vi "Dashboard Main.vi"() -> ()   [LabVIEW 2016]
uses:
  <vilib>/Utility/miscctls.llb/LVRowAndColumnTypeDef.ctl
  <vilib>/event_ctls.llb/eventvkey.ctl
  <vilib>/Rock Robotics/Network Tables/NT Write Boolean.vi
  <vilib>/Rock Robotics/Network Tables/NT Read Numeric Array.vi
  <vilib>/Rock Robotics/WPI/Dashboard/WPI_DashboardLogging Global.vi
panel:
  out "Camera Image":T1(plugin-control)
  in  "Camera Settings Right":T2={"Frame Rate"=30, "Compression"=30, "Size"=1, "DB Camera Config"=FALSE} {"Frame Rate" scale=1.0..30.0; "Compression" scale=100.0..-1.0; "Size" items=["640x480", "320x240", "160x120"]}
  in  "Camera Name Right":string(combo)="No Camera Selection"
  out "Camera Info":cluster{"Mbps LED":bool, "Mbps":dbl, "fps":dbl} {"fps" format="%#.1g"; "Mbps" format="%#.1g"}
  in  "Camera Settings":T2={"Frame Rate"=30, "Compression"=30, "Size"=1, "DB Camera Config"=FALSE} {"Frame Rate" scale=1.0..30.0; "Compression" scale=100.0..-1.0; "Size" items=["640x480", "320x240", "160x120"]}
  in  "TCP":refnum<k5>
  in  "Rec Mode":enum32{"Stop", "Record", "Playback"}(radio)
  out "Robot IP":string
  out "Image Message":string="Timeout in Camera Communications"
  in  "Dashboard Tab":T3(tab)
  in  "Select Auto":string(combo)="Select Autonomous ..."
  out "NT Connection":bool
  out "MotorChart R":cluster{"Numeric":dbl, "Numeric":dbl}(graph)
  out "MotorChart L":cluster{"Numeric":dbl, "Numeric":dbl}(graph)
  out "MotorSliders R":cluster{"MotorSlide1":dbl, "MotorSlide2":dbl} {"MotorSlide2" scale=-1.0..1.0 scale format="%#_2e"; "MotorSlide1" scale=-1.0..1.0 scale format="%#_2e"}
  out "MotorSliders L":cluster{"MotorSlide1":dbl, "MotorSlide2":dbl} {"MotorSlide2" scale=-1.0..1.0 scale format="%#_2e"; "MotorSlide1" scale=-1.0..1.0 scale format="%#_2e"}
  out "Gyro":dbl(knob) scale=0.0..360.0
  out "JS1 Z":dbl(slide) scale=-1.0..1.0 scale format="%#_2e"
  out "JS1 Graph":cluster{"X":dbl, "Y":dbl}[](graph)
  out "JS1 Buttons":T4
  out "JS2 Z":dbl(slide) scale=-1.0..1.0 scale format="%#_2e"
  out "JS2 Graph":cluster{"X":dbl, "Y":dbl}[](graph)
  out "JS2 Buttons":T4
  out "Mode":T5(ring)=enum."Auto Disabled"
  out "Camera Image Right":T1(plugin-control)
  in  "DB/String 9":string
  in  "DB/String 8":string
  in  "DB/String 7":string
  in  "DB/String 6":string
  in  "DB/String 5":string
  in  "DB/String 4":string
  in  "DB/String 3":string
  in  "DB/String 2":string
  in  "DB/String 1":string
  in  "DB/String 0":string
  in  "DB/Slider 0":dbl(slide) scale=0.0..5.0
  in  "DB/Slider 1":dbl(slide) scale=0.0..5.0
  in  "DB/Slider 2":dbl(slide) scale=0.0..5.0
  in  "DB/Slider 3":dbl(slide) scale=0.0..5.0
  out "DB/LED 3":bool
  out "DB/LED 2":bool
  out "DB/LED 1":bool
  out "DB/LED 0":bool
  in  "DB/Button 3":bool
  in  "DB/Button 2":bool
  in  "DB/Button 1":bool
  in  "DB/Button 0":bool caption="New Name"
  out "2D Picture":picture
  out "String 3 MAGIC":string
  out "Berg Mode":string
  in  "Auton Enabled":bool=TRUE
  out "String 2":string
  out "Steam Power":dbl(knob)=88.16248842081647 scale=0.0..100.0
  in  "Station Loc":T6(radio)
  out "Gyro":dbl(knob) scale=0.0..360.0
  out "Game Time":u8(slide) scale=0.1..100.0
  in  "UpdateCam":bool
  in  "Exposure":dbl(slide) scale=0.0..100.0
  in  "White Bal":dbl(slide) scale=0.0..100.0
  in  "Color Components":T7={"Hue"={110.0, 142.0}, "Sat"={212.5, 255.0}, "Val"={24.285714285714285, 112.32142857142857}, "Boolean"=FALSE} {"Val" scale=0.0..255.0; "Sat" scale=0.0..255.0; "Hue" scale=0.0..255.0 scale format="%#_3g"}
  in  "Camera Mode":u16(ring) items=["Raw", "Interpreted", "Particle", "Paired", "Final"]
  in  "Color Components 2":T7={"Hue"={110.0, 142.0}, "Sat"={212.0, 255.0}, "Val"={24.0, 112.0}, "Boolean"=FALSE} {"Val" scale=0.0..255.0; "Sat" scale=0.0..255.0; "Hue" scale=0.0..255.0 scale format="%#_3g"}
  in  "Camera Mode 2":u16(ring) items=["Raw", "Interpreted", "Particle", "Paired", "Final"]
  in  "Test Slider":dbl(slide) scale=0.0..100.0 scale format="%#_3g"
  in  "On/Off":bool caption="Solenoid"
  in  "Test Name":u16(ring) items=["Select the test to run..."]
  in  "Test Tree":string(tree)
  in  "Motor":cluster{"Value":dbl, "Enable":bool} {"Value" scale=-1.0..1.0 scale format="%#_3g"}
  out "Progress":T8 {"Test Progress" scale=0.0..100.0}
  in  "Rev/Fwd":cluster{"Forward":bool, "Reverse":bool}
  in  "Test Ring":u16(ring) items=["Monochrome", "Color"]
  out "Cmd Status":string
  in  "Execute Command":bool
  in  "Command Params":string[][](table)
  in  "Command Selection":i32(listbox)
  in  "CheckList":i32(listbox)
  out "Tree":string(tree)
  out "Background":bool
  in  "Camera Name":string(combo)="No Camera Selection"
  # "HW"
  # "HW"
  # "Joysticks"
  # "Drive Motors"
  # "Front"
  # "Right"
  # "Left"
  # "Back"
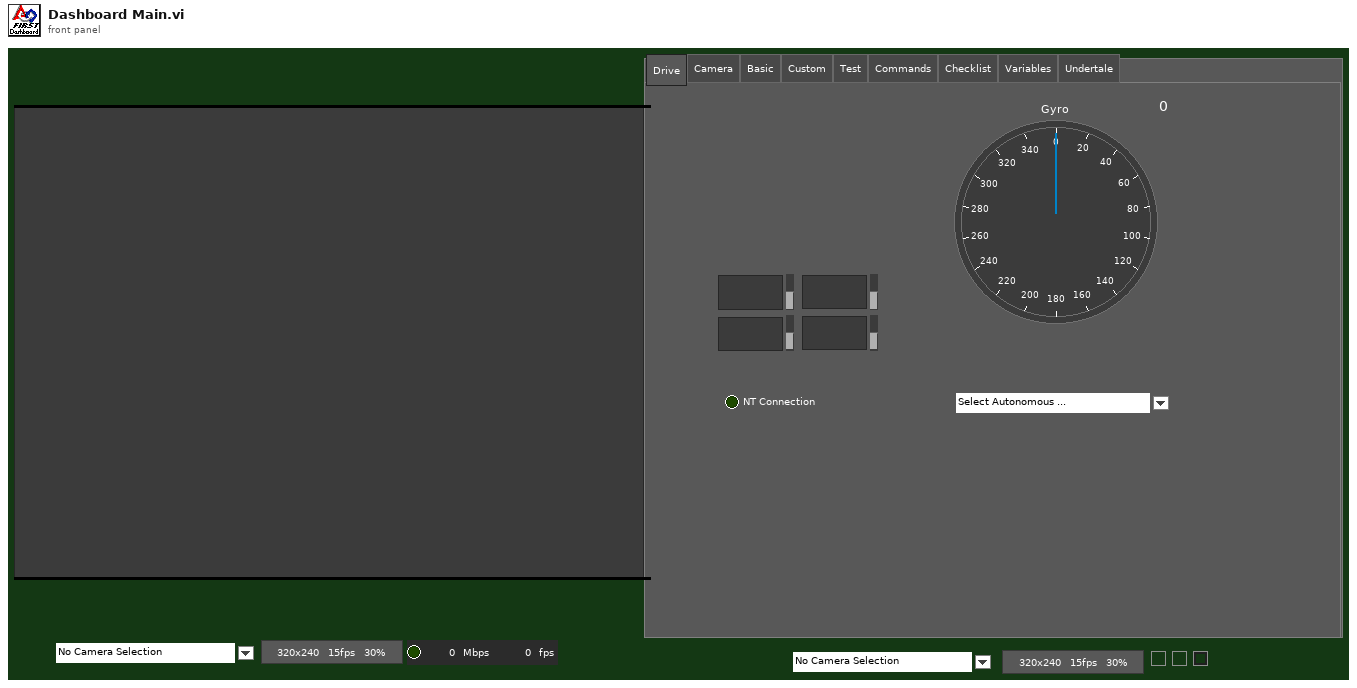
[diagram p1: front panel]
types:
  T1 = typedef "IMAQ Image.ctl" = refnum<image>
  T2 = cluster{"Frame Rate":i32, "Compression":i32, "Size":u16, "DB Camera Config":bool}
  T3 = enum32{"Drive", "Camera", "Basic", "Custom", "Test", "Commands", "Checklist", "Variables", "Undertale"}
  T4 = cluster{bool, bool, bool, bool, bool, bool, bool, bool, bool, bool, bool, bool}
  T5 = enum8{"Tele-Op Disabled", "Tele-Op Enabled", "Auto Disabled", "Auto Enabled", "Test Disabled", "Test Enabled", "Disconnected", "No Code", "E-Stop"}
  T6 = enum32{"Radio Selection 1", "Radio Selection 2", "Radio Selection 3"}
  T7 = cluster{"Hue":cluster{dbl, dbl}, "Sat":cluster{dbl, dbl}, "Val":cluster{dbl, dbl}, "Boolean":bool}
  T8 = cluster{"Test Progress":u8, "Test Progress Text":string}
  T9 = typedef "Image Type" = u32
  T10 = cluster{"IDs":cluster{"RPC field ID":u16, "Unique ID":u16}, "String":string}
  T11 = enum32{"Drive", "Basic", "Custom", "Test", "Checklist", "Variables"}
  T12 = cluster{"Error Strings":string, "Disable Counts":cluster{u16, u16}, "Rail Faults":cluster{u16, u16, u16}, "Robot IP":string, "DB Mode":u8, "Event Info":cluster{"Name":string, "Type":u8, "Number":u16, "Replay":u8}}
  T13 = cluster{"Storage":cluster{"Disk Free":u64, "RAM Block":u32, "RAM free":u32}, "CPU Utilization":cluster{"CPU % ISR":sgl, "CPU % Time Crit":sgl, "CPU % Timed Str":sgl, "CPU % High":sgl, "CPU % Above":sgl, "CPU % Normal":sgl, "CPU % Low":sgl}, "CAN":cluster{"% Bus Utilization":sgl, "Bus Off Cnt":u32, "TX_FIFO Full Cnt":u32, "Receive Error Cnt":u8, "Transmit Error Cnt":u8}, "HID":cluster{"HID Outputs":u32, "Rumble Low":u16, "Rumble High":u16}[]}
  T14 = cluster{"Status bits":cluster{"Test Mode":bool, "Autonomous":bool, "Enabled":bool, "Code Start":bool, "Brownout":bool, "Reserved 2":bool, "Reserved 3":bool, "E-Stop":bool}, "Code Trace":cluster{"Disabled":bool, "TeleOp":bool, "Auto":bool, "Test":bool}, "Controller Type":enum16{"unknown", "cRIO", "roboRio"}, "Code?":enum16{"unknown", "noCode", "code"}, "Battery V":dbl}
  T15 = cluster{"Control Bits":cluster{"TestMode":bool, "Autonomous":bool, "Enabled":bool, "FMS Present":bool, bool, bool, bool, "E-Stop":bool}, "Team Station ":u8, "Countdown":sgl, "Joystick Values":cluster{"Axes":dbl[], "Buttons":bool[], "POVs":i16[]}[]}
  T16 = cluster{"Axes":dbl[], "Buttons":bool[], "POVs":i16[]}[]
  T17 = cluster{"Axes":dbl[], "Buttons":bool[], "POVs":i16[]}
  T18 = cluster{"Buttons[0]":bool, "Buttons[1]":bool, "Buttons[2]":bool, "Buttons[3]":bool, "Buttons[4]":bool, "Buttons[5]":bool, "Buttons[6]":bool, "Buttons[7]":bool, "Buttons[8]":bool, "Buttons[9]":bool, "Buttons[10]":bool, "Buttons[11]":bool}
  T19 = cluster{"Camera Image":refnum<vi>, "Dashboard Tab":refnum<vi>, "Background":refnum<vi>, "Rec Mode":refnum<vi>, "Test Slider":refnum<vi>, "On/Off ":refnum<vi>, "Test Ring":refnum<vi>, "Rev/Fwd":refnum<vi>, "Test Name":refnum<vi>, "Motor":refnum<vi>, "Progress":refnum<vi>, "CheckList":refnum<vi>, "Tree":refnum<vi>, "Test Tree":refnum<vi>, "Command Params":refnum<vi>, "Command Selection":refnum<vi>, "Execute Command":refnum<vi>, "Cmd Status":refnum<vi>, "Camera Settings":refnum<vi>, "Camera Name":refnum<vi>, "Camera Info":refnum<vi>, "Camera Settings Right":refnum<vi>, "Camera Name Right":refnum<vi>, "Camera Image Right":refnum<vi>}
  T20 = cluster{"Target Combined":cluster{"Particle Report":cluster{"Area":dbl, "Number of Holes":dbl, "Bounding Rect":cluster{"Left":dbl, "Top":dbl, "Right":dbl, "Bottom":dbl}, "Center of Mass":cluster{"X":dbl, "Y":dbl}, "Orientation":dbl, "Dimensions":cluster{"Width":dbl, "Height":dbl}}, "Aspect Ratio Score":dbl, "Vertical Hollowness":dbl, "Horizontal Hollowness":dbl}, "Target A":cluster{"Particle Report":cluster{"Area":dbl, "Number of Holes":dbl, "Bounding Rect":cluster{"Left":dbl, "Top":dbl, "Right":dbl, "Bottom":dbl}, "Center of Mass":cluster{"X":dbl, "Y":dbl}, "Orientation":dbl, "Dimensions":cluster{"Width":dbl, "Height":dbl}}, "Aspect Ratio Score":dbl, "Vertical Hollowness":dbl, "Horizontal Hollowness":dbl}, "Target B":cluster{"Particle Report":cluster{"Area":dbl, "Number of Holes":dbl, "Bounding Rect":cluster{"Left":dbl, "Top":dbl, "Right":dbl, "Bottom":dbl}, "Center of Mass":cluster{"X":dbl, "Y":dbl}, "Orientation":dbl, "Dimensions":cluster{"Width":dbl, "Height":dbl}}, "Aspect Ratio Score":dbl, "Vertical Hollowness":dbl, "Horizontal Hollowness":dbl}}
  T21 = cluster{"Particle Report":cluster{"Area":dbl, "Number of Holes":dbl, "Bounding Rect":cluster{"Left":dbl, "Top":dbl, "Right":dbl, "Bottom":dbl}, "Center of Mass":cluster{"X":dbl, "Y":dbl}, "Orientation":dbl, "Dimensions":cluster{"Width":dbl, "Height":dbl}}, "Aspect Ratio Score":dbl, "Vertical Hollowness":dbl, "Horizontal Hollowness":dbl}
  T22 = cluster{"Operation":enum16{"Update", "Clear"}, "Color Box":u32}[]
  T23 = typedef "eventvkey.ctl" = enum16{"ASCII", "Enter", "Return", "Shift", "Ctrl", "Alt", "Cmd", "Opt", "Caps", "NumLock", "Clear", "Break", "Up", "Down", "Left", "Right", "Insert", "Delete", "Home", "End", "PageUp", "PageDown", "Escape", "Help", "Pause", "ScrollLock", "F1", "F2", "F3", "F4", "F5", "F6", "F7", "F8", "F9", "F10", "F11", "F12", "F13", "F14", "F15", "F16", "F17", "F18", "F19", "F20", "F21", "F22", "F23", "F24", "Play", "VolumeUp", "VolumeDown", "Mute", "Two Byte Char"}
  T24 = cluster{"Image Size":bool, "Image Type":bool, "Pixel Value":bool, "ROI Information":bool, "Zoom Factor":bool}
  T25 = cluster{"Operation":enum16{"Update", "Clear"}, "Color Box":u32}
  T26 = typedef "LVRowAndColumnTypeDef.ctl" = cluster{"Row":i32, "Column":i32}
  T27 = cluster{"Shift":bool, "Ctrl":bool, "Alt":bool, "Cmd":bool, "Opt":bool}
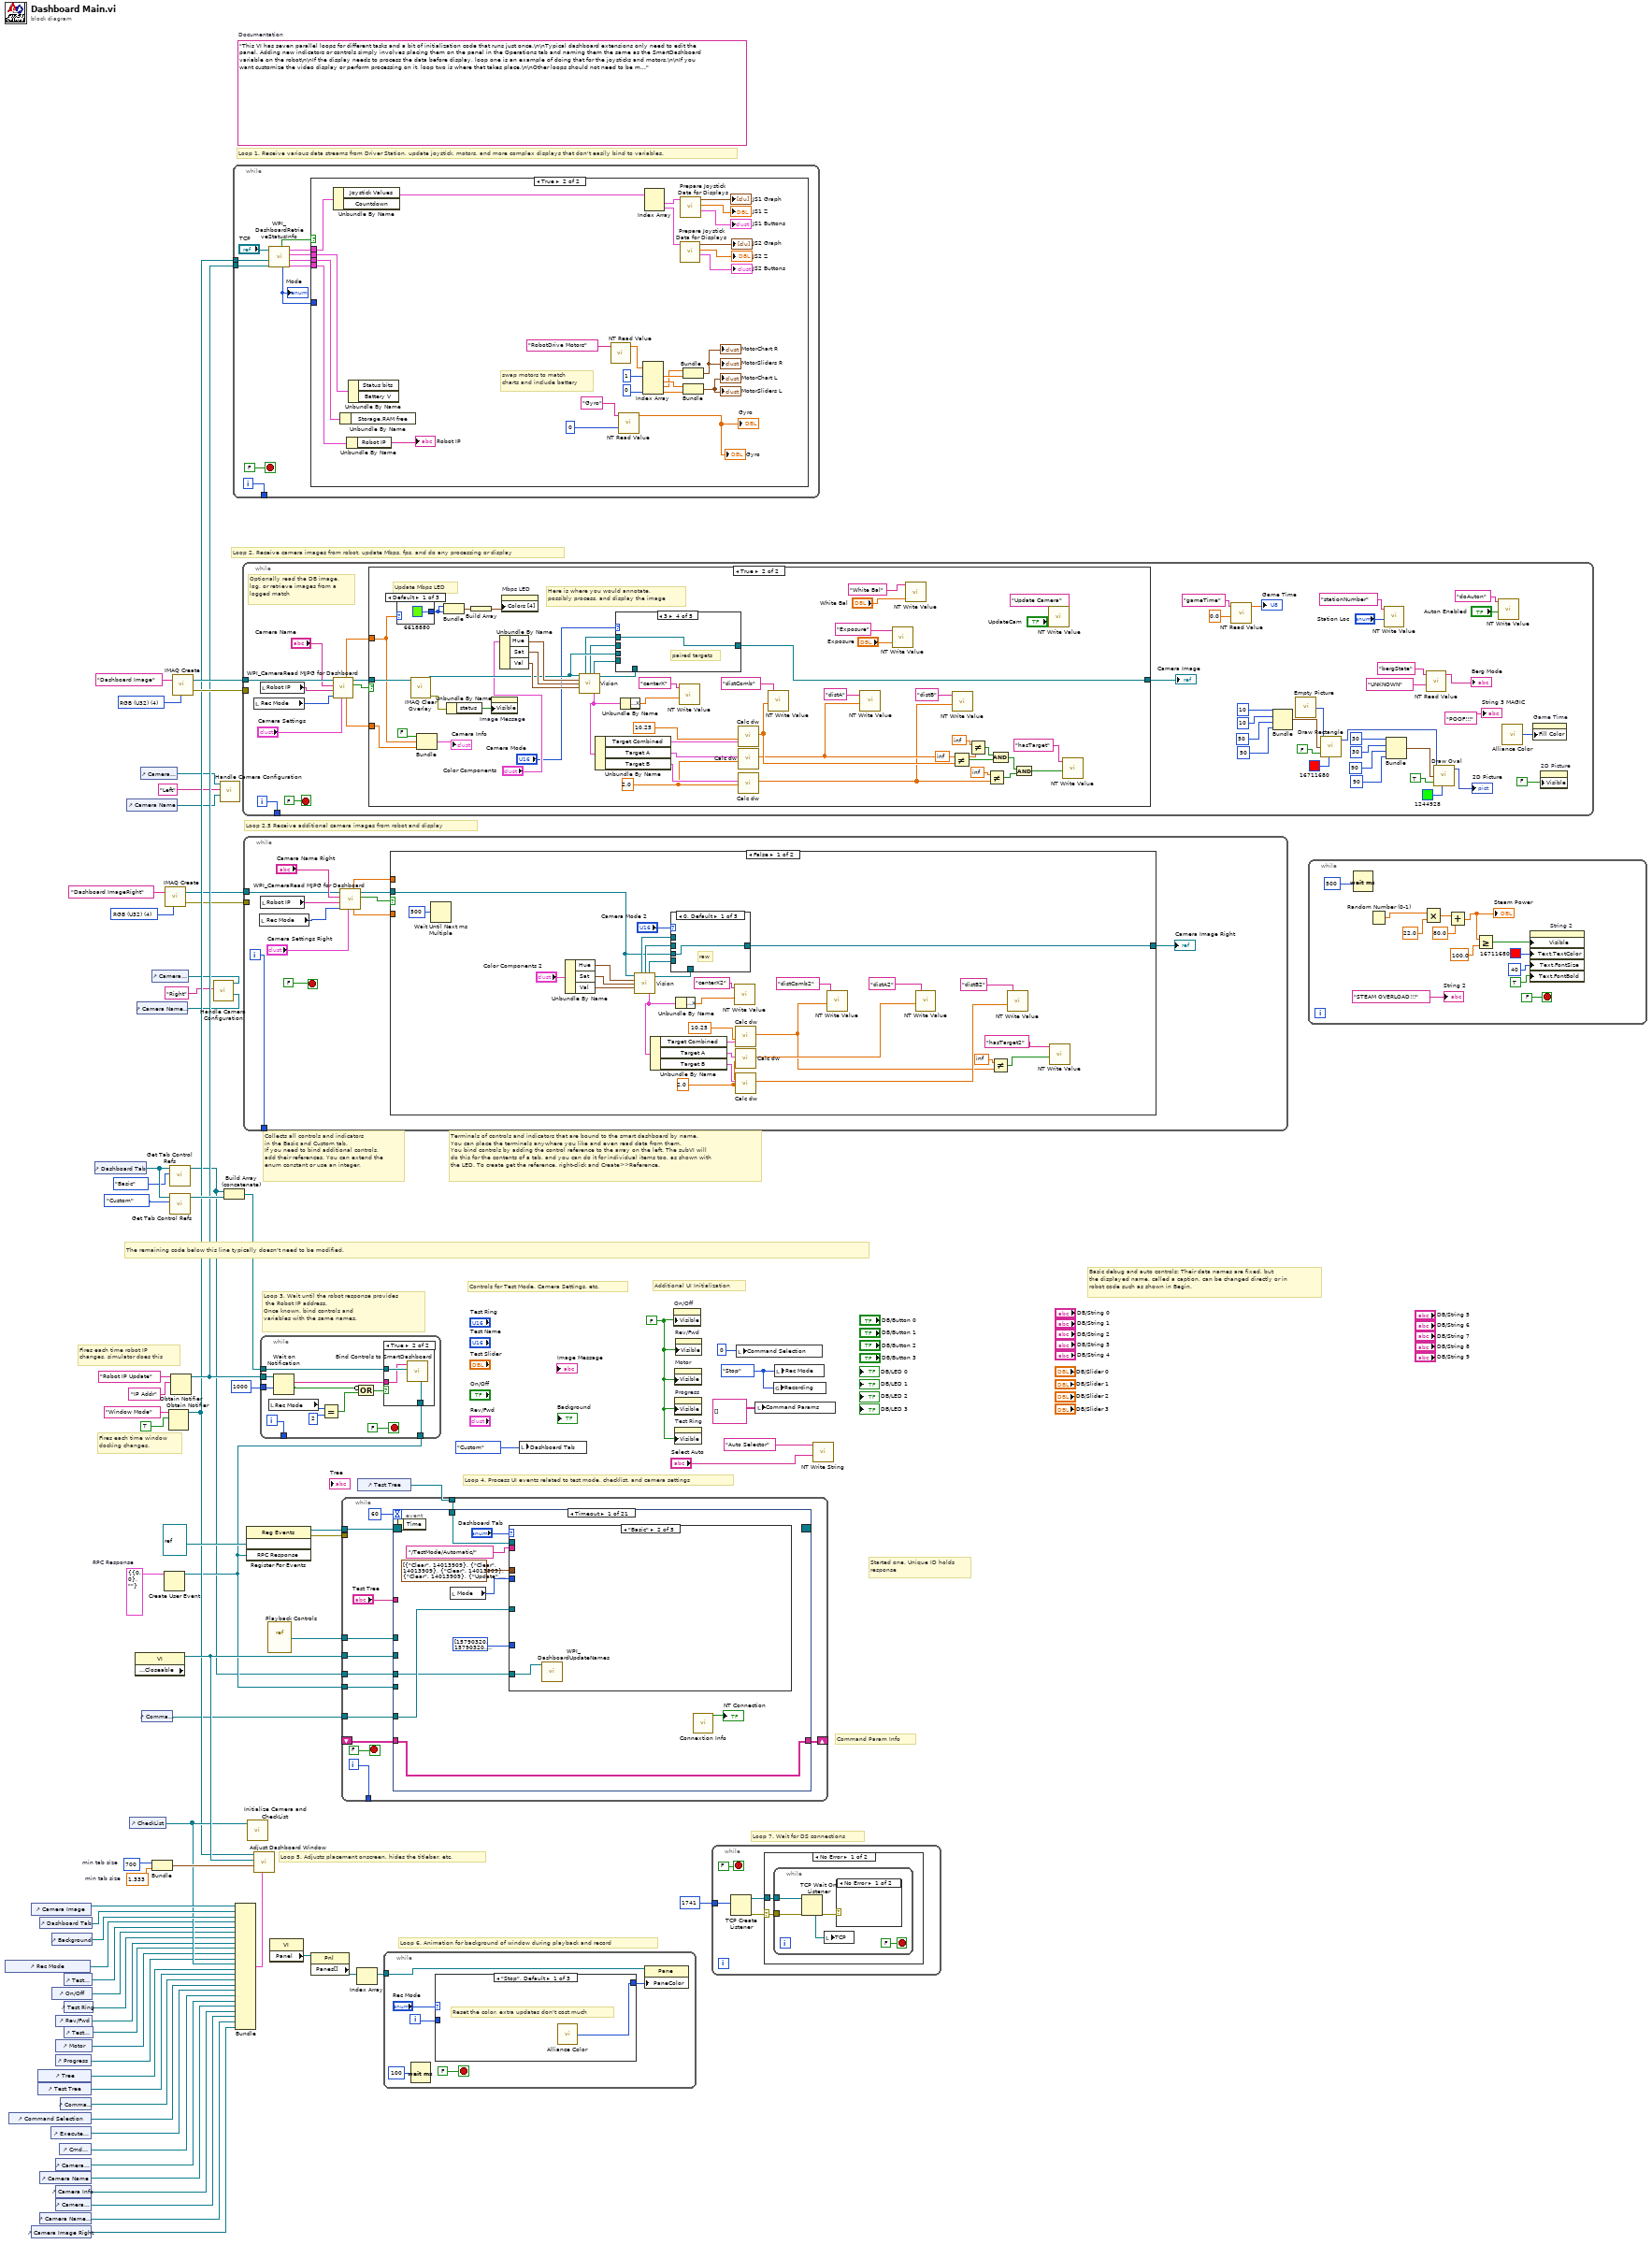
[diagram p0: block diagram]
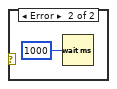
[diagram p7: hidden frame]
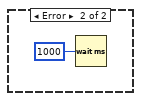
[diagram p8: hidden frame]
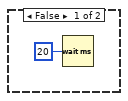
[diagram p9: hidden frame]
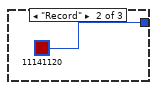
[diagram p10: hidden frame]
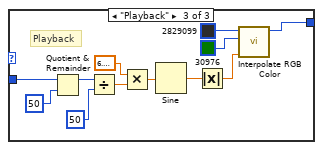
[diagram p11: hidden frame]
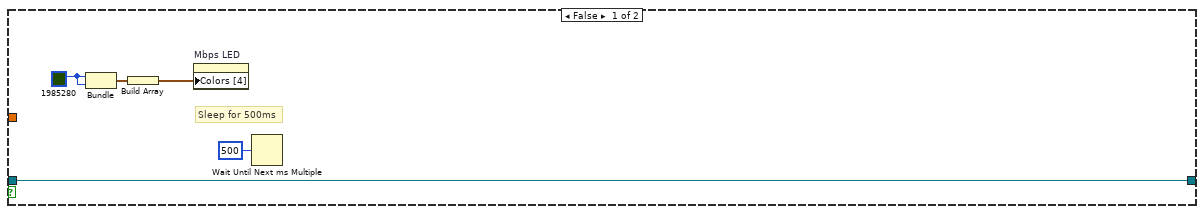
[diagram p13: hidden frame]
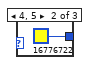
[diagram p18: hidden frame]
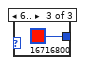
[diagram p19: hidden frame]
diagram:
  w10 = T9 4 items=["Grayscale (U8)", "Grayscale (I16)", "Grayscale (SGL)", "Complex (CSG)", "RGB (U32)", "HSL (U32)", "RGB (U64)"] ("Image Type")
  w26 = T10 {"IDs"={"RPC field ID"=0, "Unique ID"=0}, "String"=""}  # RPC Response
  w51 = 700  # min tab size
  w50 = 1.333  # min tab size
  w58 = enum32{"Stop", "Record", "Playback"}."Stop" ("Rec Mode")
  w33 = FALSE ("Visible")
  (unwired) "This VI has seven parallel loops for different tasks and a bit of initialization code that runs just once.\n\nTypical dashboard extensions only need to edit the panel. Adding new indicators or controls simply involves placing them on the panel in the Operations tab and naming them the same as the SmartDashboard variable on the robot\n\nIf the display needs to process the data before display, loop one is an example of doing that for the joysticks and motors.\n\nIf you want customize the video display or perform processing on it, loop two is where that takes place.\n\nOther loops should not need to be modified. They are pretty standard, and document the task they perform."  # Documentation
  w75 = T9 4 items=["Grayscale (U8)", "Grayscale (I16)", "Grayscale (SGL)", "Complex (CSG)", "RGB (U32)", "HSL (U32)", "RGB (U64)"] ("Image Type")
  # "Loop 2.5 Receive additional camera images from robot and display"
  # "Command Param Info"
  # "Started one, Unique ID holds\nresponse"
  # "Loop 7. Wait for DS connections"
  # "Basic debug and auto controls: Their data names are fixed, but\nthe displayed name, called a caption, can be changed directly or in\nrobot code such as shown in Begin."
  # "Controls for Test Mode, Camera Settings, etc."
  # "Additional UI Initialization"
  # "Loop 6. Animation for background of window during playback and record"
  # "Fires each time robot IP\nchanges, simulator does this"
  # "Fires each time window\ndocking changes."
  # "Collects all controls and indicators\nin the Basic and Custom tab.\nIf you need to bind additional controls,\nadd their references. You can extend the\nenum constant or use an integer."
  # "The remaining code below this line typically doesn't need to be modified."
  # "Loop 4. Process UI events related to test mode, checklist, and camera settings"
  # "Terminals of controls and indicators that are bound to the smart dashboard by name.\nYou can place the terminals anywhere you like and even read data from them.\nYou bind controls by adding the control reference to the array on the left. The subVI will\ndo this for the contents of a tab, and you can do it for individual items too, as shown with\nthe LED. To create get the reference, right-click and Create>>Reference."
  # "Loop 3. Wait until the robot response provides\n the Robot IP address.\nOnce known, bind controls and\nvariables with the same names."
  # "Loop 5. Adjusts placement onscreen, hides the titlebar, etc."
  # "Loop 1. Receive various data streams from Driver Station, update joystick, motors, and more complex displays that don't easily bind to variables."
  # "Loop 2. Receive camera images from robot, update Mbps, fps, and do any processing or display"
  n1 = control-ref of="Rec Mode"() -> (w39:refnum<vi>)
  n2 = control-ref of="Command Selection"() -> (w25:refnum<vi>)
  n3 = control-ref of="Camera Image Right"() -> (w1:refnum<vi>)
  n4 = control-ref of="Camera Image"() -> (w53:refnum<vi>)
  n5 = control-ref of="Tree"() -> (w43:refnum<vi>)
  n6 = control-ref of="Test Tree"() -> (w42:refnum<vi>)
  n7 = control-ref of="Dashboard Tab"() -> (w52:refnum<vi>)
  n8 = control-ref of="Camera Name"() -> (w16:refnum<vi>)
  n9 = control-ref of="Camera Name Right"() -> (w2:refnum<vi>)
  n10 = control-ref of="Execute Command"() -> (w27:refnum<vi>)
  n11 = control-ref of="Background"() -> (w48:refnum<vi>)
  n12 = control-ref of="On/Off"() -> (w37:refnum<vi>)
  n13 = control-ref of="Progress"() -> (w34:refnum<vi>)
  n14 = control-ref of="Camera Settings"() -> (w17:refnum<vi>)
  n15 = control-ref of="Camera Info"() -> (w15:refnum<vi>)
  n16 = control-ref of="Camera Settings Right"() -> (w3:refnum<vi>)
  n17 = control-ref of="Rev/Fwd"() -> (w35:refnum<vi>)
  n18 = control-ref of="Motor"() -> (w40:refnum<vi>)
  n19 = control-ref of="Cmd Status"() -> (w21:refnum<vi>)
  n20 = control-ref of="Command Params"() -> (w28:refnum<vi>)
  n21 = control-ref of="Test Slider"() -> (w38:refnum<vi>)
  n22 = control-ref of="Test Ring"() -> (w36:refnum<vi>)
  n23 = control-ref of="Test Name"() -> (w41:refnum<vi>)
  n24 = control-ref of="Dashboard Tab"() -> (w56:refnum<vi>)
  n25 = control-ref of="Camera Name"() -> (w18:refnum<vi>)
  n26 = control-ref of="CheckList"() -> (w44:refnum<vi>)
  n27 = property class="VI" props=["Front Panel.Closeable"]() -> (reference out=w57:refnum<vi>)  [unwired: 2 in, 2 out]
  n28 = control-ref of="Camera Name Right"() -> (w6:refnum<vi>)
  n29 = control-ref of="Camera Settings"() -> (w19:refnum<vi>)
  n30 = control-ref of="Command Params"() -> (w20:refnum<vi>)
  n31 = control-ref of="Camera Settings Right"() -> (w7:refnum<vi>)
  n32 = Bundle("min tab size"=w51, "min tab size"=w50) -> (w49:cluster{"min tab size":i32, "min tab size":dbl})  [unwired: 1 in]
  n33 = Create User Event(user event datatype=w26) -> (user event=w22:refnum<user-event>)  [unwired: 1 in, 1 out]
  n34 = call "IMAQ Create"("Image Name"="Dashboard ImageRight", "Image Type"=w10) -> ("New Image"=w9:T1, "error out"=w8:errorcluster)  [unwired: 2 in, 1 out]
  n35 = Obtain Notifier(name (unnamed)="Window Mode", notification data type=TRUE) -> (notifier out=w31:refnum<notifier>)  [unwired: 2 in, 2 out]
  n36 = call <vilib>:"Get Tab Control Refs.vi"("Page Index"=T11."Basic" ("Dashboard Tab"), "TabControl in"=w56) -> ("ControlsOnPage"=w14:refnum<vi>[])  [unwired: 9 in]
  n37 = call <vilib>:"Get Tab Control Refs.vi"("Page Index"=T11."Custom" ("Dashboard Tab"), "TabControl in"=w56) -> ("ControlsOnPage"=w55:refnum<vi>[])  [unwired: 9 in]
  n38 = Obtain Notifier(name (unnamed)="Robot IP Update", notification data type="IP Addr" ("name (unnamed)")) -> (notifier out=w32:refnum<notifier>)  [unwired: 2 in, 2 out]
  n39 = call "IMAQ Create"("Image Name"="Dashboard Image", "Image Type"=w75) -> ("New Image"=w73:T1, "error out"=w72:errorcluster)  [unwired: 2 in, 1 out]
  n40 = call "Handle Camera Configuration.vi"("CameraNameRef"=w6, "Camera File Name"="Right", "ClusterRef"=w7) -> ()  [unwired: 9 in]
  n41 = call "Handle Camera Configuration.vi"("CameraNameRef"=w18, "Camera File Name"="Left", "ClusterRef"=w19) -> ()  [unwired: 9 in]
  n42 = Build Array (concatenate)(w14, w55) -> (w54:refnum<vi>[])
  n43 = while {
    tunnel: [w85] -> _
    tunnel: w32 -> [w79]
    tunnel: w31 -> [w76]
    i -> [w85]
    stop <- FALSE stop-if-true
    n44 = call <vilib>:"WPI_DashboardRetrieveStatusInfo.vi"("Binding Refnum"=w79, "Window Mode Notifier"=w76, "TCP Cnx"="TCP") -> ("Power and Errors"=w80:T12, "Robot Metrics"=w83:T13, "Status Info"=w84:T14, "Control Info"=w81:T15, "Robot Mode"=w78:T5, "Process?"=w82:bool)  [unwired: 3 in]
    "Mode" <- w78
    n45 = case shown="True" w82 {
      tunnel: w84 -> [_ w114]
      tunnel: w83 -> [_ w113]
      tunnel: w81 -> [_ w112]
      tunnel: w80 -> [_ w111]
      tunnel: w78 -> [_ _]
      frame False {
        n46 = Wait (ms)(milliseconds to wait=u32 20) -> ()  [unwired: 1 out]
      }
      frame True {
        # "swap motors to match\ncharts and include battery"
        n47 = Unbundle By Name(w112) -> ("Joystick Values"=w102:T16)  [unwired: 1 out]
        n48 = Unbundle By Name(w113) -> ()  [unwired: 1 out]
        n49 = Unbundle By Name(w111) -> ("Robot IP"=→"Robot IP":string)
        n50 = Unbundle By Name(w114) -> ()  [unwired: 2 out]
        n51 = call-poly <vilib>:"NT Read Value.vi"("Name"="RobotDrive Motors") -> ("Numeric Array"=w92:dbl[])  [unwired: 9 in, 1 out]
        n52 = call-poly <vilib>:"NT Read Value.vi"("Default Value"=0, "Name"="Gyro") -> ("Numeric"=→"Gyro" →"Gyro":dbl)  [unwired: 8 in, 1 out]
        n53 = Index Array(array=w92, index #1=1, index #4=0) -> (element #1=w106:dbl, element #2=w107:dbl, element #3=w105:dbl, element #4=w110:dbl)  [unwired: 2 in]
        n54 = Index Array(array=w102) -> (element #1=w101:T17, element #2=w97:T17)  [unwired: 2 in]
        n55 = call "Prepare Joystick Data for Displays.vi"("Joystick Values"=w97) -> ("Buttons"=→"JS2 Buttons":T18, "Z Axis"=→"JS2 Z":dbl, "Cartesian Data"=→"JS2 Graph":cluster{"X axis":dbl, "X axis":dbl}[])  [unwired: 8 in]
        n56 = call "Prepare Joystick Data for Displays.vi"("Joystick Values"=w101) -> ("Buttons"=→"JS1 Buttons":T18, "Z Axis"=→"JS1 Z":dbl, "Cartesian Data"=→"JS1 Graph":cluster{"X axis":dbl, "X axis":dbl}[])  [unwired: 8 in]
        n57 = Bundle("Numeric"=w105, "Numeric"=w106) -> (→"MotorChart R" →"MotorSliders R":cluster{"Numeric":dbl, "Numeric":dbl})  [unwired: 1 in]
        n58 = Bundle("Numeric"=w107, "Numeric"=w110) -> (→"MotorChart L" →"MotorSliders L":cluster{"Numeric":dbl, "Numeric":dbl})  [unwired: 1 in]
      }
    }
  }
  n59 = Bundle("Camera Image"=w53, "Dashboard Tab"=w52, "Background"=w48, "Rec Mode"=w39, "Test Slider"=w38, "On/Off"=w37, "Test Ring"=w36, "Rev/Fwd"=w35, "Test Name"=w41, "Motor"=w40, "Progress"=w34, "CheckList"=w44, "Tree"=w43, "Test Tree"=w42, "Command Params"=w28, "Command Selection"=w25, "Execute Command"=w27, "Cmd Status"=w21, "Camera Settings"=w17, "Camera Name"=w16, "Camera Info"=w15, "Camera Settings Right"=w3, "Camera Name Right"=w2, "Camera Image Right"=w1) -> (w45:T19)  [unwired: 1 in]
  n60 = while {
    tunnel: w73 -> [w154]
    tunnel: w72 -> [_]
    tunnel: [w155] -> _
    i -> [w155]
    stop <- FALSE stop-if-true
    # "Optionally read the DB image,\nlog, or retrieve images from a\nlogged match"
    n61 = local read "Rec Mode"() -> (w150:enum32{"Stop", "Record", "Playback"})
    n62 = local read "Robot IP"() -> (w149:string)
    n63 = call <vilib>:"WPI_CameraRead MJPG for Dashboard.vi"("Camera Settings"="Camera Settings", "Rec Mode"=w150, "Robot IP"=w149, "Camera Name"="Camera Name", "Refnum in"=w154) -> ("Active"=w152:bool, "Refnum out"=w153:T1, "FPS"=w151:dbl, "Bandwidth (Mbps)"=w148:dbl)  [unwired: 3 in]
    n64 = case shown="True" w152 {
      tunnel: w153 -> [w157 w207]
      tunnel: w148 -> [_ w204]
      tunnel: w151 -> [_ w205]
      tunnel: [w157 w196] -> w145
      frame False {
        w159 = u32 1985280 ("Color Box")
        # "Sleep for 500ms"
        n65 = Bundle("Color Box"=w159, "Color Box"=w159) -> (w160:cluster{"Color Box":u32, "Color Box":u32})  [unwired: 1 out]
        n66 = Build Array(w160) -> (w158:cluster{"Color Box":u32, "Color Box":u32}[])
        n67 = property on="Mbps LED" class="Bool (strict)"("Colors [4]"=w158) -> ()  [unwired: 2 in, 2 out]
        n68 = Wait Until Next ms Multiple(millisecond multiple=u32 500) -> ()  [unwired: 1 out]
      }
      frame True {
        w182 = 2.0
        # "Here is where you would annotate,\npossibly process, and display the image"
        # "Update Mbps LED"
        n69 = case shown="Default" w204 {
          tunnel: [u32 6618880 ("Color Box") u32 16776722 ("Color Box") u32 16716800 ("Color Box")] -> w208
          frame Default {
          }
          frame 4, 5 {
          }
          frame 6.. {
          }
        }
        n70 = call "IMAQ Clear Overlay"("Image"=w207) -> ("error out"=w210:errorcluster, "Image Out"=w197:T1)  [unwired: 2 in, 7 out]
        n71 = Bundle(FALSE, "Bandwidth (Mbps)"=w204, "FPS"=w205) -> (→"Camera Info":cluster{bool, "Bandwidth (Mbps)":dbl, "FPS":dbl})  [unwired: 1 in]
        n72 = Bundle("Color Box"=w208, "Color Box"=w208) -> (w209:cluster{"Color Box":u32, "Color Box":u32})  [unwired: 1 out]
        n73 = Unbundle By Name(w210) -> ("status"=w211:bool)
        n74 = Build Array(w209) -> (w206:cluster{"Color Box":u32, "Color Box":u32}[])
        n75 = property on="Image Message" class="Str"("Visible"=w211) -> ()  [unwired: 2 in, 2 out]
        n76 = Unbundle By Name("Color Components") -> ("Hue"=w200:cluster{dbl, dbl}, "Sat"=w199:cluster{dbl, dbl}, "Val"=w198:cluster{dbl, dbl})
        n77 = property on="Mbps LED" class="Bool (strict)"("Colors [4]"=w206) -> ()  [unwired: 2 in, 2 out]
        n78 = call "Vision.vi"("Image In"=w197, "Hue Range"=w200, "Sat Range"=w199, "Luma Range"=w198) -> ("Particle Out Paired"=w192:T1, "Particle Out"=w194:T1, "Thresholded Out"=w195:T1, "Final Out"=w193:T1, "Out"=w190:T20)  [unwired: 7 in]
        n79 = Unbundle By Name(w190) -> ("Target Combined"=w189:T21, "Target A"=w185:T21, "Target B"=w184:T21)
        n80 = case shown="3" "Camera Mode" {
          tunnel: w197 -> [w212 _ _ _ _]
          tunnel: [w212 w213 w214 w215 w216] -> w196
          tunnel: w195 -> [_ w213 _ _ _]
          tunnel: w194 -> [_ _ w214 _ _]
          tunnel: w193 -> [_ _ _ _ w216]
          tunnel: w192 -> [_ _ _ w215 _]
          frame 0, Default {
            # "raw"
          }
          frame 1 {
            # "interpreted"
          }
          frame 2 {
            # "particle"
          }
          frame 3 {
            # "paired targets"
          }
          frame 4 {
            # "final"
          }
        }
        n81 = Unbundle By Name(w190) -> ("Target Combined.Particle Report.Center of Mass.X"=w191:dbl)
        n82 = call-poly <vilib>:"NT Write Value.vi"("Numeric"=w191, "Name"="centerX") -> ()  [unwired: 9 in, 1 out]
        n83 = call "Calc dw.vi"("Width T in incheees"=10.25, "Target"=w189) -> ("dw"=w179:dbl)  [unwired: 9 in]
        n84 = call "Calc dw.vi"("Width T in incheees"=w182, "Target"=w185) -> ("dw"=w165:dbl)  [unwired: 9 in]
        n85 = call "Calc dw.vi"("Width T in incheees"=w182, "Target"=w184) -> ("dw"=w164:dbl)  [unwired: 9 in]
        n86 = call-poly <vilib>:"NT Write Value.vi"("Numeric"=w179, "Name"="distComb") -> ()  [unwired: 9 in, 1 out]
        n87 = call-poly <vilib>:"NT Write Value.vi"("Numeric"=w165, "Name"="distA") -> ()  [unwired: 9 in, 1 out]
        n88 = call-poly <vilib>:"NT Write Value.vi"("Numeric"="Exposure", "Name"="Exposure") -> ()  [unwired: 9 in, 1 out]
        n89 = call-poly <vilib>:"NT Write Value.vi"("Numeric"="White Bal", "Name"="White Bal") -> ()  [unwired: 9 in, 1 out]
        n90 = Not Equal?(x=inf, y=w179) -> (x != y?=w169:bool)
        n91 = call-poly <vilib>:"NT Write Value.vi"("Numeric"=w164, "Name"="distB") -> ()  [unwired: 9 in, 1 out]
        n92 = Not Equal?(x=inf, y=w165) -> (x != y?=w170:bool)
        n93 = Not Equal?(x=inf, y=w164) -> (x != y?=w168:bool)
        n94 = And(x=w170, y=w169) -> (x .and. y?=w167:bool)
        n95 = And(x=w167, y=w168) -> (x .and. y?=w166:bool)
        n96 = call-poly <vilib>:"NT Write Value.vi"("Boolean"="UpdateCam", "Name"="Update Camera") -> ()  [unwired: 9 in, 1 out]
        n97 = call-poly <vilib>:"NT Write Value.vi"("Boolean"=w166, "Name"="hasTarget") -> ()  [unwired: 9 in, 1 out]
      }
    }
    "Camera Image" <- w145
    n98 = call-poly <vilib>:"NT Read Value.vi"("Default Value"=0.0, "Name"="gameTime") -> ("Numeric"=→"Game Time":dbl)  [unwired: 8 in, 1 out]
    n99 = Bundle(10, 10, 50, 50) -> (w132:cluster{i32, i32, i32, i32})  [unwired: 1 in]
    n100 = call "Empty Picture"() -> ("empty picture"=w130:picture)
    n101 = call <vilib>:"Draw Rectangle.vi"("picture"=w130, "rect"=w132, "fill?(F)"=FALSE, "color(black)"=u32 16711680) -> ("new picture"=w118:picture)  [unwired: 5 in]
    n102 = call-poly <vilib>:"NT Write Value.vi"("Numeric"="Station Loc", "Name"="stationNumber") -> ()  [unwired: 9 in, 1 out]
    n103 = Bundle(30, 30, 90, 90) -> (w121:cluster{i32, i32, i32, i32})  [unwired: 1 in]
    n104 = call-poly <vilib>:"NT Read Value.vi"("Default Value"="UNKNOWN", "Name"="bergState") -> ("String"=→"Berg Mode":string)  [unwired: 8 in, 1 out]
    n105 = call <vilib>:"Draw Oval.vi"("picture"=w118, "rect"=w121, "fill?(F)"=TRUE, "color(black)"=u32 1244928) -> ("new picture"=→"2D Picture":picture)  [unwired: 5 in]
    n106 = call-poly <vilib>:"NT Write Value.vi"("Boolean"="Auton Enabled", "Name"="doAuton") -> ()  [unwired: 9 in, 1 out]
    n107 = call "Alliance Color.vi"() -> ("Alliance Color"=w144:u32)
    n108 = property on="Game Time" class="Slide (strict)"("Fill Color"=w144) -> ()  [unwired: 2 in, 2 out]
    n109 = property on="2D Picture" class="Pict"("Visible"=FALSE) -> ()  [unwired: 2 in, 2 out]
    "String 3 MAGIC" <- "POOF!!!"
  }
  n110 = while {
    tunnel: w9 -> [w230]
    tunnel: w8 -> [_]
    tunnel: [w224] -> _
    i -> [w224]
    stop <- FALSE stop-if-true
    n111 = local read "Rec Mode"() -> (w228:enum32{"Stop", "Record", "Playback"})
    n112 = local read "Robot IP"() -> (w229:string)
    n113 = call <vilib>:"WPI_CameraRead MJPG for Dashboard.vi"("Camera Settings"="Camera Settings Right", "Rec Mode"=w228, "Robot IP"=w229, "Camera Name"="Camera Name Right", "Refnum in"=w230) -> ("Active"=w223:bool, "Refnum out"=w226:T1, "FPS"=w221:dbl, "Bandwidth (Mbps)"=w222:dbl)  [unwired: 3 in]
    n114 = case shown="False" w223 {
      tunnel: w226 -> [w235 w266]
      tunnel: w222 -> [_ _]
      tunnel: w221 -> [_ _]
      tunnel: [w234 w266] -> w220
      frame False {
        w240 = 2.0
        n115 = Wait Until Next ms Multiple(millisecond multiple=u32 500) -> ()  [unwired: 1 out]
        n116 = Unbundle By Name("Color Components 2") -> ("Hue"=w258:cluster{dbl, dbl}, "Sat"=w257:cluster{dbl, dbl}, "Val"=w256:cluster{dbl, dbl})
        n117 = call "Vision.vi"("Image In"=w235, "Hue Range"=w258, "Sat Range"=w257, "Luma Range"=w256) -> ("Particle Out Paired"=w252:T1, "Particle Out"=w254:T1, "Thresholded Out"=w255:T1, "Final Out"=w253:T1, "Out"=w250:T20)  [unwired: 7 in]
        n118 = Unbundle By Name(w250) -> ("Target Combined"=w249:T21, "Target A"=w245:T21, "Target B"=w244:T21)
        n119 = case shown="0, Default" "Camera Mode 2" {
          tunnel: w235 -> [w261 _ _ _ _]
          tunnel: [w261 w262 w263 w264 w265] -> w234
          tunnel: w255 -> [_ w262 _ _ _]
          tunnel: w254 -> [_ _ w263 _ _]
          tunnel: w253 -> [_ _ _ _ w265]
          tunnel: w252 -> [_ _ _ w264 _]
          frame 0, Default {
            # "raw"
          }
          frame 1 {
            # "interpreted"
          }
          frame 2 {
            # "particle"
          }
          frame 3 {
            # "paired targets"
          }
          frame 4 {
            # "final"
          }
        }
        n120 = Unbundle By Name(w250) -> ("Target Combined.Particle Report.Center of Mass.X"=w251:dbl)
        n121 = call-poly <vilib>:"NT Write Value.vi"("Numeric"=w251, "Name"="centerX2") -> ()  [unwired: 9 in, 1 out]
        n122 = call "Calc dw.vi"("Width T in incheees"=10.25, "Target"=w249) -> ("dw"=w237:dbl)  [unwired: 9 in]
        n123 = call "Calc dw.vi"("Width T in incheees"=w240, "Target"=w245) -> ("dw"=w243:dbl)  [unwired: 9 in]
        n124 = call "Calc dw.vi"("Width T in incheees"=w240, "Target"=w244) -> ("dw"=w242:dbl)  [unwired: 9 in]
        n125 = call-poly <vilib>:"NT Write Value.vi"("Numeric"=w237, "Name"="distComb2") -> ()  [unwired: 9 in, 1 out]
        n126 = call-poly <vilib>:"NT Write Value.vi"("Numeric"=w243, "Name"="distA2") -> ()  [unwired: 9 in, 1 out]
        n127 = Not Equal?(x=inf, y=w237) -> (x != y?=w236:bool)
        n128 = call-poly <vilib>:"NT Write Value.vi"("Numeric"=w242, "Name"="distB2") -> ()  [unwired: 9 in, 1 out]
        n129 = call-poly <vilib>:"NT Write Value.vi"("Boolean"=w236, "Name"="hasTarget2") -> ()  [unwired: 9 in, 1 out]
      }
      frame True {
      }
    }
    "Camera Image Right" <- w220
  }
  n130 = register-events(refnum<vi> refnum, w22) -> (reference out=w62:refnum<event-registration>, error out=w61:errorcluster)  [unwired: 2 in]
  n131 = call "Initialize Camera and CheckList.vi"("ListBox in"=w44) -> ()  [unwired: 11 in]
  n132 = call "Adjust Dashboard Window.vi"("Sizing Refnums"=w45, "Size Constraints"=w49, "VI"=w57, "WIn Mode"=w31) -> ()  [unwired: 8 in]
  n133 = while {
    tunnel: w54 -> [w278]
    tunnel: w32 -> [w276]
    tunnel: [w274] -> _
    tunnel: u32 1000 ("milliseconds to wait") -> [w273]
    tunnel: w22 -> [w267]
    i -> [w274]
    stop <- FALSE stop-if-true
    n134 = local read "Rec Mode"() -> (w269:enum32{"Stop", "Record", "Playback"})
    n135 = Wait on Notification(notifier=w276, timeout in ms (-1)=w273) -> (notification=w275:string, timed out?=w271:bool)  [unwired: 2 in, 2 out]
    n136 = Equal?(x=w269, y=u16 2 ("Rec Mode")) -> (x = y?=w270:bool)
    n137 = Compound Arithmetic op=OR(invert w271, w270) -> (w272:bool)
    n138 = case shown="True" w272 {
      tunnel: w278 -> [_ w281]
      tunnel: w275 -> [_ w280]
      tunnel: w267 -> [_ w279]
      frame False {
      }
      frame True {
        n139 = call <vilib>:"Bind Controls to SmartDashboard.vi"("RPC ref"=w279, "Bound Control Refs"=w281, "Server IP Address"=w280) -> ()  [unwired: 9 in]
      }
    }
  }
  n140 = vi-ref "Playback Controls.vi"() -> (w63:refnum<vi>)
  n141 = property class="VI"() -> ("Panel"=w65:refnum<vi>)  [unwired: 2 in, 2 out]
  n142 = property class="Pnl"(reference=w65) -> ("Panes[]"=w66:refnum<vi>[])  [unwired: 1 in, 2 out]
  n143 = Index Array(array=w66) -> (element=w64:refnum<vi>)  [unwired: 1 in]
  n144 = control-ref of="Test Tree"() -> (w67:refnum<vi>)
  n145 = while {
    tunnel: [w291] -> _
    tunnel: w67 -> [w290]
    tunnel: w63 -> [w289]
    tunnel: w62 -> [w288]
    tunnel: w61 -> [_]
    tunnel: w57 -> [w287]
    tunnel: w22 -> [w286]
    tunnel: w20 -> [w285]
    shift-right: [w284] -> _
    shift-left: _ -> [w283]
    tunnel: w14 -> [w282]
    i -> [w291]
    stop <- FALSE stop-if-true
    n146 = event shown="[0] Timeout" {
      selector: w288 -> [_ _ _ _ _ _ _ _ _ _ _ _ _ _ _ _ _ _ _ _ _]
      dyn-events: [_ _ _ _ _ _ _ _ _ _ _ _ _ _ _ _ w547 _ _ _ _] -> _
      timeout: u32 60 ("milliseconds to wait") -> [_ _ _ _ _ _ _ _ _ _ _ _ _ _ _ _ _ _ _ _ _]
      tunnel: w290 -> [w303 _ _ _ _ _ _ _ _ _ _ _ _ _ _ _ _ _ _ _ _]
      tunnel: "Test Tree" -> [_ _ _ _ _ _ _ _ _ _ _ w514 w522 w524 w528 w536 _ _ _ _ _]
      tunnel: w289 -> [_ _ _ _ _ _ _ _ _ _ _ _ _ _ _ _ w549 _ w567 _ _]
      tunnel: w287 -> [_ _ _ _ _ _ _ _ _ _ _ _ _ _ _ _ w545 _ _ _ _]
      tunnel: w286 -> [_ _ _ _ _ _ _ _ _ _ _ _ _ _ _ _ w541 _ _ _ _]
      tunnel: w285 -> [w298 _ _ _ _ _ w465 _ _ _ _ _ _ _ _ _ _ _ _ _ _]
      tunnel: [w297 w342 w444 w449 w458 w462 w463 w472 w482 w489 w501 w513 w520 w523 w527 w535 w540 w562 w564 w568 w579] -> w284
      tunnel: w283 -> [w297 w342 w444 w449 w458 w462 w463 _ _ w489 w501 w513 w520 w523 w527 w535 w540 w562 w564 w568 w579]
      tunnel: w282 -> [w295 _ _ _ _ _ _ _ _ _ _ _ _ _ _ _ _ _ _ _ _]
      event Timeout {
        n147 = event-data() -> ()  [unwired: 1 in, 1 out]
        n148 = local read "Mode"() -> (w300:T5)
        n149 = case shown="\"Basic\"" "Dashboard Tab" {
          tunnel: w303 -> [_ _ w319 _ _]
          tunnel: "/TestMode/Automatic/" ("Name Pattern") -> [_ _ w318 _ _]
          tunnel: T22 [{"Operation"=enum."Clear", "Color Box"=14013909}, {"Operation"=enum."Clear", "Color Box"=14013909}, {"Operation"=enum."Clear", "Color Box"=14013909}, {"Operation"=enum."Clear", "Color Box"=14013909}, {"Operation"=enum."Update", "Color Box"=14013909}, {"Operation"=enum."Update", "Color Box"=16777215}, {"Operation"=enum."Clear", "Color Box"=14013909}, {"Operation"=enum."Clear", "Color Box"=14013909}, {"Operation"=enum."Clear", "Color Box"=14013909}] -> [_ _ w311 _ w335]
          tunnel: w300 -> [_ _ w310 _ w334]
          tunnel: u32[] [15790320, 15790320, 15790320, 15790320, 16777215, 16777215, 15790320, 15790320, 15790320] -> [_ _ _ _ w340]
          tunnel: w298 -> [_ _ _ _ w328]
          tunnel: w295 -> [_ w305 _ _ _]
          frame "Custom", Default {
          }
          frame "Basic" {
            n150 = call <vilib>:"WPI_DashboardUpdateNames.vi"("Controls on Tab"=w305) -> ()  [unwired: 11 in]
          }
          frame "Test" {
            w317 = -2 ("Active Item:Row Number")
            n151 = Index Array(array=w311, index=w310) -> (element=w312:T25)
            n152 = Unbundle(w312) -> ("Operation"=w313:enum16{"Update", "Clear"}, "Color Box"=w314:u32)
            n153 = call <vilib>:"NT Read String.vi"("Name"="/TestMode/TestName") -> ("String"=w308:string)  [unwired: 9 in, 1 out]
            n154 = call <vilib>:"NT Read and Format Entries as Tree.vi"("Operation"=w313, "Name Pattern"=w318, "Tree Refnum"=w319) -> ()  [unwired: 7 in, 2 out]
            n155 = case shown="\"\"" w308 {
              tunnel: "/TestMode/TestProgress" ("Name") -> [w321 _]
              tunnel: "/TestMode/TestProgressText" ("Name") -> [w320 _]
              frame Default {
                n156 = call <vilib>:"NT Read Number.vi"("Name"=w321) -> ("Numeric"=w322:dbl)  [unwired: 9 in, 1 out]
                n157 = call <vilib>:"NT Read String.vi"("Name"=w320) -> ("String"=w323:string)  [unwired: 9 in, 1 out]
                n158 = Bundle("Numeric"=w322, "String"=w323) -> (→"Progress":cluster{"Numeric":dbl, "String":string})  [unwired: 1 in]
              }
              frame "" {
                n159 = property on="Progress" class="Clust (strict)"("Visible"=FALSE) -> ()  [unwired: 2 in, 2 out]
                n160 = local write "Test Name"(u16 0) -> ()
              }
            }
            n161 = property on="Test Tree" class="Tree (strict)"("Active Item Row Number"=w317, "ActiveColNum"=w317, "CellBG"=w314, "Active Item Row Number"=-1 ("Active Item:Row Number"), "CellBG"=u32 5789784 ("Color Box")) -> ()  [unwired: 2 in, 2 out]
          }
          frame "Variables" {
            n162 = control-ref of="Tree"() -> (w327:refnum<vi>)
            n163 = call <vilib>:"NT Read and Format Entries as Tree.vi"("Tree Refnum"=w327) -> ()  [unwired: 9 in, 2 out]
          }
          frame "Commands" {
            w336 = u32 5789784 ("Color Box")
            w337 = T26 {"Row"=-1, "Column"=-2} ("Active Cell:Active Cell")
            w339 = T26 {"Row"=-2, "Column"=-2} ("Active Cell:Active Cell")
            n164 = Index Array(array=w340, index=w334) -> (element=w338:u32)
            n165 = Index Array(array=w335, index=w334) -> (element=w333:T25)
            n166 = Unbundle(w333) -> ("Operation"=w332:enum16{"Update", "Clear"})  [unwired: 1 out]
            n167 = local read "Command Selection"() -> (w331:i32)
            n168 = property on="Command Selection" class="MCListbox (strict)"("ActiveCell"=w339, "CellBG"=w338, "ActiveCell"=w337, "CellBG"=w336) -> ()  [unwired: 2 in, 2 out]
            n169 = call <vilib>:"WPI_DashboardUpdate RPC Info.vi"("Operation"=w332) -> ("update"=w330:bool, "commands"=w329:string[][])  [unwired: 9 in]
            n170 = property on="Command Selection" class="MCListbox (strict)"("ItemNames"=w329) -> ()  [unwired: 2 in, 2 out]
            n171 = property on="Command Params" class="Tbl (strict)"("Active Cell"=w339, "Cell BG Color"=w338, "Active Cell"=w337, "Cell BG Color"=w336) -> ()  [unwired: 2 in, 2 out]
            n172 = call <vilib>:"WPI_DashboardUpdate Command Params.vi"("Update"=w330, "NewVal"=w331, "Commands"=w329, "Param Tbl"=w328) -> ()  [unwired: 7 in, 1 out]
          }
        }
        n173 = call <vilib>:"Connextion Info.vi"() -> ("Connected"=→"NT Connection":bool)  [unwired: 10 in, 1 out]
      }
      event "Test Tree": Value Change {
        # "Show appropriate\ncontrols"
        n174 = event-data() -> ("CtlRef"=w345:refnum<vi>, "NewVal"=w343:string)  [unwired: 1 in]
        n175 = call <vilib>:"WPI_UtilitiesGetTreeIOName.vi"("NewVal"=w343, "TreeControl in"=w345) -> ("I/O Name"=w346:string)  [unwired: 9 in]
        n176 = case shown="\"Camera\"" w346 {
          selector: w346 -> [_ w353 _ w375 w384 _]
          tunnel: w343 -> [_ _ w372 w374 _ w391]
          tunnel: cluster{string[]}[] [{["640x480", "320x240", "160x120"]}, {["Auto", "Fixed indoor", "Fixed outdoor 1", "Fixed outdoor 2", "Fixed fluorescent 1", "Fixed fluorescent 2", "Hold current"]}, {["Auto", "Flicker-free 50 Hz", "Flicker-free 60 Hz", "Hold current"]}, {["None", "Prioritize frame rate", "Prioritize image quality"]}, {["Monochrome", "Color"]}] -> [_ _ _ _ _ w390]
          frame Default {
            w348 = FALSE ("Visible")
            w347 = FALSE ("Visible")
            n177 = property on="Motor" class="Clust (strict)"("Visible"=w347) -> ()  [unwired: 2 in, 2 out]
            n178 = property on="Test Ring" class="Ring (strict)"("Visible"=w347) -> ()  [unwired: 2 in, 2 out]
            n179 = property on="Rev/Fwd" class="Clust (strict)"("Visible"=w348) -> ()  [unwired: 2 in, 2 out]
            n180 = property on="On/Off" class="Bool (strict)"("Visible"=w348) -> ()  [unwired: 2 in, 2 out]
            n181 = property on="Test Slider" class="Slide (strict)"("Visible"=w348) -> ()  [unwired: 2 in, 2 out]
          }
          frame "Analog Out", "Motor", "PWM" {
            w354 = FALSE ("Visible")
            n182 = case shown="\"Analog Out\"" w353 {
              tunnel: [1.0 ("Value") -1.0 ("Value") 0.0 ("Value")] -> w352
              tunnel: [255.0 ("Value") 1.0 ("Value") 5.0 ("Value")] -> w351
              tunnel: [128.0 ("Value") 0.0 ("Value") 0.0 ("Value")] -> w350
              tunnel: [64.0 ("Value") 0.5 ("Value") 1.0 ("Value")] -> w349
              frame "PWM" {
              }
              frame "Motor", Default {
              }
              frame "Analog Out" {
              }
            }
            n183 = property on="Motor" class="Clust (strict)"("Visible"=TRUE) -> ()  [unwired: 2 in, 2 out]
            n184 = property on="Value" class="Slide (strict)"("Value"=w350, "Scale.Minimum"=w352, "Scale.Maximum"=w351, "Scale.Increment"=w349) -> ()  [unwired: 2 in, 2 out]
            n185 = property on="On/Off" class="Bool (strict)"("Visible"=w354) -> ()  [unwired: 2 in, 2 out]
            n186 = property on="Test Slider" class="Slide (strict)"("Visible"=w354) -> ()  [unwired: 2 in, 2 out]
            n187 = property on="Test Ring" class="Ring (strict)"("Visible"=w354) -> ()  [unwired: 2 in, 2 out]
            n188 = property on="Rev/Fwd" class="Clust (strict)"("Visible"=w354) -> ()  [unwired: 2 in, 2 out]
          }
          frame "Servo" {
            w370 = FALSE ("Visible")
            n189 = call <vilib>:"NT Read Number.vi"("Name"=w372) -> ("Numeric"=w371:dbl)  [unwired: 9 in, 1 out]
            n190 = property on="Test Slider" class="Slide (strict)"("Visible"=TRUE, "Scale.Maximum"=170.0 ("Scale.Range:Maximum")) -> ()  [unwired: 2 in, 2 out]
            n191 = local write "Test Slider"(w371) -> ()
            n192 = property on="Motor" class="Clust (strict)"("Visible"=w370) -> ()  [unwired: 2 in, 2 out]
            n193 = property on="Rev/Fwd" class="Clust (strict)"("Visible"=w370) -> ()  [unwired: 2 in, 2 out]
            n194 = property on="On/Off" class="Bool (strict)"("Visible"=w370) -> ()  [unwired: 2 in, 2 out]
            n195 = property on="Test Ring" class="Ring (strict)"("Visible"=w370) -> ()  [unwired: 2 in, 2 out]
          }
          frame "Relay", "Solenoid" {
            w373 = FALSE ("Visible")
            n196 = property on="Motor" class="Clust (strict)"("Visible"=w373) -> ()  [unwired: 2 in, 2 out]
            n197 = property on="Test Slider" class="Slide (strict)"("Visible"=w373) -> ()  [unwired: 2 in, 2 out]
            n198 = Search and Replace String(input string=w374, search string="/Value  **", replace string="/Direction") -> (result string=w380:string)  [unwired: 5 in, 3 out]
            n199 = property on="Test Ring" class="Ring (strict)"("Visible"=w373) -> ()  [unwired: 2 in, 2 out]
            n200 = call <vilib>:"NT Read String.vi"("Name"=w380) -> ("String"=w378:string)  [unwired: 9 in, 1 out]
            n201 = Equal?(x="Both directions", y=w378) -> (x = y?=w376:bool)
            n202 = Not(x=w376) -> (.not. x?=w377:bool)
            n203 = property on="Rev/Fwd" class="Clust (strict)"("Visible"=w376) -> ()  [unwired: 2 in, 2 out]
            n204 = property on="On/Off" class="Bool (strict)"("Visible"=w377, "Caption.Text"=w375) -> ()  [unwired: 2 in, 2 out]
          }
          frame "Compressor", "Digital Out" {
            w383 = FALSE ("Visible")
            # "Get direction and finish"
            n205 = property on="Motor" class="Clust (strict)"("Visible"=w383) -> ()  [unwired: 2 in, 2 out]
            n206 = property on="Test Slider" class="Slide (strict)"("Visible"=w383) -> ()  [unwired: 2 in, 2 out]
            n207 = property on="Test Ring" class="Ring (strict)"("Visible"=w383) -> ()  [unwired: 2 in, 2 out]
            n208 = property on="On/Off" class="Bool (strict)"("Visible"=TRUE, "Caption.Text"=w384) -> ()  [unwired: 2 in, 2 out]
            n209 = property on="Rev/Fwd" class="Clust (strict)"("Visible"=FALSE) -> ()  [unwired: 2 in, 2 out]
          }
          frame "Camera" {
            n210 = call <vilib>:"Get Last Path Segment.vi"("String in"=w391) -> ("String out"=w392:string)  [unwired: 10 in]
            n211 = property on="On/Off" class="Bool (strict)"("Visible"=FALSE) -> ()  [unwired: 2 in, 2 out]
            n212 = property on="Motor" class="Clust (strict)"("Visible"=FALSE) -> ()  [unwired: 2 in, 2 out]
            n213 = property on="Rev/Fwd" class="Clust (strict)"("Visible"=FALSE) -> ()  [unwired: 2 in, 2 out]
            n214 = case shown="\"White Balance  **\"" w392 {
              tunnel: w391 -> [w398 w407 w416 w425 w434 _ w440]
              tunnel: w390 -> [w396 w404 w413 w422 w431 _ _]
              frame "Size  **" {
                n215 = Index Array(array=w396) -> (element=w395:cluster{string[]})  [unwired: 1 in]
                n216 = call <vilib>:"NT Read String.vi"("Name"=w398) -> ("String"=w397:string)  [unwired: 9 in, 1 out]
                n217 = Unbundle(w395) -> (w393:string[])
                n218 = Match First String(2:w393, 3:w397) -> (0:w394:i32)  [unwired: 1 out]
                n219 = property on="Test Ring" class="Ring (strict)"("Value"=w394, "Strings []"=w393) -> ()  [unwired: 2 in, 2 out]
                n220 = property on="Test Ring" class="Ring (strict)"("Visible"=TRUE) -> ()  [unwired: 2 in, 2 out]
                n221 = property on="Test Slider" class="Slide (strict)"("Visible"=FALSE) -> ()  [unwired: 2 in, 2 out]
              }
              frame "White Balance  **" {
                n222 = Index Array(array=w404, index=1) -> (element=w405:cluster{string[]})
                n223 = call <vilib>:"NT Read String.vi"("Name"=w407) -> ("String"=w406:string)  [unwired: 9 in, 1 out]
                n224 = Unbundle(w405) -> (w402:string[])
                n225 = Match First String(2:w402, 3:w406) -> (0:w401:i32)  [unwired: 1 out]
                n226 = property on="Test Ring" class="Ring (strict)"("Value"=w401, "Strings []"=w402) -> ()  [unwired: 2 in, 2 out]
                n227 = property on="Test Ring" class="Ring (strict)"("Visible"=TRUE) -> ()  [unwired: 2 in, 2 out]
                n228 = property on="Test Slider" class="Slide (strict)"("Visible"=FALSE) -> ()  [unwired: 2 in, 2 out]
              }
              frame "Exposure  **" {
                n229 = Index Array(array=w413, index=2) -> (element=w414:cluster{string[]})
                n230 = call <vilib>:"NT Read String.vi"("Name"=w416) -> ("String"=w415:string)  [unwired: 9 in, 1 out]
                n231 = Unbundle(w414) -> (w410:string[])
                n232 = Match First String(2:w410, 3:w415) -> (0:w411:i32)  [unwired: 1 out]
                n233 = property on="Test Ring" class="Ring (strict)"("Value"=w411, "Strings []"=w410) -> ()  [unwired: 2 in, 2 out]
                n234 = property on="Test Ring" class="Ring (strict)"("Visible"=TRUE) -> ()  [unwired: 2 in, 2 out]
                n235 = property on="Test Slider" class="Slide (strict)"("Visible"=FALSE) -> ()  [unwired: 2 in, 2 out]
              }
              frame "Exposure Priority  **" {
                n236 = Index Array(array=w422, index=3) -> (element=w423:cluster{string[]})
                n237 = call <vilib>:"NT Read String.vi"("Name"=w425) -> ("String"=w424:string)  [unwired: 9 in, 1 out]
                n238 = Unbundle(w423) -> (w419:string[])
                n239 = Match First String(2:w419, 3:w424) -> (0:w420:i32)  [unwired: 1 out]
                n240 = property on="Test Ring" class="Ring (strict)"("Value"=w420, "Strings []"=w419) -> ()  [unwired: 2 in, 2 out]
                n241 = property on="Test Ring" class="Ring (strict)"("Visible"=TRUE) -> ()  [unwired: 2 in, 2 out]
                n242 = property on="Test Slider" class="Slide (strict)"("Visible"=FALSE) -> ()  [unwired: 2 in, 2 out]
              }
              frame "Color Enable  **" {
                n243 = Index Array(array=w431, index=4) -> (element=w432:cluster{string[]})
                n244 = call <vilib>:"NT Read String.vi"("Name"=w434) -> ("String"=w433:string)  [unwired: 9 in, 1 out]
                n245 = Unbundle(w432) -> (w428:string[])
                n246 = Match First String(2:w428, 3:w433) -> (0:w429:i32)  [unwired: 1 out]
                n247 = property on="Test Ring" class="Ring (strict)"("Value"=w429, "Strings []"=w428) -> ()  [unwired: 2 in, 2 out]
                n248 = property on="Test Ring" class="Ring (strict)"("Visible"=TRUE) -> ()  [unwired: 2 in, 2 out]
                n249 = property on="Test Slider" class="Slide (strict)"("Visible"=FALSE) -> ()  [unwired: 2 in, 2 out]
              }
              frame Default {
                n250 = property on="Test Ring" class="Ring (strict)"("Visible"=FALSE) -> ()  [unwired: 2 in, 2 out]
                n251 = property on="Test Slider" class="Slide (strict)"("Visible"=FALSE) -> ()  [unwired: 2 in, 2 out]
              }
              frame "Brightness  **", "Color Level  **", "Compression  **", "FPS  **", "Sharpness  **" {
                n252 = call <vilib>:"NT Read Number.vi"("Name"=w440) -> ("Numeric"=w439:dbl)  [unwired: 9 in, 1 out]
                n253 = local write "Test Slider"(w439) -> ()
                n254 = property on="Test Slider" class="Slide (strict)"("Visible"=TRUE, "Scale.Maximum"=100.0 ("Scale.Range:Maximum")) -> ()  [unwired: 2 in, 2 out]
                n255 = property on="Test Ring" class="Ring (strict)"("Visible"=FALSE) -> ()  [unwired: 2 in, 2 out]
              }
            }
          }
        }
        n256 = property on="Progress" class="Clust (strict)"("Visible"=FALSE) -> ()  [unwired: 2 in, 2 out]
      }
      event "Test Name": Mouse Enter {
        # "Populate the ring with the list of tests"
        n257 = event-data() -> ()  [unwired: 1 in, 1 out]
        n258 = call <vilib>:"NT Read String Array.vi"("Name"="/TestMode/TestList") -> ("String Array"=w448:string[])  [unwired: 9 in, 1 out]
        n259 = Build Array (concatenate)("Select the test to run...", w448) -> (w447:string[])
        n260 = property on="Test Name" class="Ring (strict)"("Strings []"=w447) -> ()  [unwired: 2 in, 2 out]
      }
      event "Test Name": Value Change {
        w450 = FALSE ("Visible")
        # "Tell the robot the test name to run"
        n261 = event-data() -> ("NewVal"=w454:u16)  [unwired: 1 in]
        n262 = property on="Test Name" class="Ring (strict)"() -> ("Strings []"=w455:string[])  [unwired: 2 in, 2 out]
        n263 = local write "Progress"(T8 {"Test Progress"=0, "Test Progress Text"=""} ("Progress")) -> ()
        n264 = Index Array(array=w455, index=w454) -> (element=w453:string)
        n265 = call <vilib>:"NT Write String.vi"("String"=w453, "Name"="/TestMode/TestName") -> ()  [unwired: 9 in, 1 out]
        n266 = property on="Progress" class="Clust (strict)"("Visible"=TRUE) -> ()  [unwired: 2 in, 2 out]
        n267 = property on="Motor" class="Clust (strict)"("Visible"=w450) -> ()  [unwired: 2 in, 2 out]
        n268 = property on="Test Slider" class="Slide (strict)"("Visible"=w450) -> ()  [unwired: 2 in, 2 out]
        n269 = property on="On/Off" class="Bool (strict)"("Visible"=w450) -> ()  [unwired: 2 in, 2 out]
        n270 = property on="Rev/Fwd" class="Clust (strict)"("Visible"=w450) -> ()  [unwired: 2 in, 2 out]
        n271 = property on="Test Ring" class="Ring (strict)"("Visible"=w450) -> ()  [unwired: 2 in, 2 out]
      }
      event "Select Auto": Mouse Enter {
        # "Populate the combo box with the list of autonomous options"
        n272 = event-data() -> ()  [unwired: 1 in, 1 out]
        n273 = call <vilib>:"NT Read String Array.vi"("Name"="Auto List") -> ("String Array"=w457:string[])  [unwired: 9 in, 1 out]
        n274 = property on="Select Auto" class="CmbBox"("Strings[]"=w457) -> ()  [unwired: 2 in, 2 out]
      }
      event "Select Auto": Value Change {
        # "User modified the Auto Selection. Write to NT variable so robot knows."
        n275 = event-data() -> ("NewVal"=w460:string)  [unwired: 1 in]
        n276 = call <vilib>:"NT Write String.vi"("String"=w460, "Name"="Auto Selector") -> ()  [unwired: 9 in, 1 out]
      }
      event "Command Selection": Value Change {
        # "Get the params and show in table"
        n277 = event-data() -> ("NewVal"=w466:i32)  [unwired: 1 in]
        n278 = property on="Command Selection" class="MCListbox (strict)"() -> ("ItemNames"=w464:string[][])  [unwired: 2 in, 2 out]
        n279 = call <vilib>:"WPI_DashboardUpdate Command Params.vi"("NewVal"=w466, "Commands"=w464, "Param Tbl"=w465) -> ()  [unwired: 8 in, 1 out]
      }
      event "Execute Command": Value Change {
        # "Started one, Unique ID holds\nresponse"
        n280 = event-data() -> ()  [unwired: 1 in, 1 out]
        n281 = property on="Command Selection" class="MCListbox (strict)"() -> ("ItemNames"=w477:string[][])  [unwired: 2 in, 2 out]
        n282 = Index Array(array=w477, index (row)="Command Selection", index (col)=0) -> (element=w475:string)
        n283 = call <vilib>:"Invoke Commands.vi"("Command Params"="Command Params", "Function Name"=w475) -> ("Params"=w471:u8, "Started"=w470:bool)  [unwired: 7 in, 1 out]
        n284 = Array Subset(array="Command Params", length (row)=w471) -> (w472:string[][])  [unwired: 3 in]
        n285 = Select(t="Executing" ("Cmd Status"), s=w470, f="" ("Cmd Status")) -> (s? t:f=→"Cmd Status":string)
      }
      event "Command Selection": Double Click {
        n286 = event-data() -> ("Row"=w485:i32)  [unwired: 1 in]
        n287 = property on="Command Selection" class="MCListbox (strict)"() -> ("ItemNames"=w488:string[][])  [unwired: 2 in, 2 out]
        n288 = local read "Command Params"() -> (w484:string[][])
        n289 = Index Array(array=w488, index (row)=w485, index (col)=0) -> (element=w486:string)
        n290 = call <vilib>:"Invoke Commands.vi"("Command Params"=w484, "Function Name"=w486) -> ("Params"=w483:u8, "Started"=w478:bool)  [unwired: 7 in, 1 out]
        n291 = Array Subset(array=w484, length (row)=w483) -> (w482:string[][])  [unwired: 3 in]
        n292 = Select(t="Executing" ("Cmd Status"), s=w478, f="" ("Cmd Status")) -> (s? t:f=w479:string)
        n293 = local write "Cmd Status"(w479) -> ()
      }
      event "CheckList": Double Click {
        # "Shift clears all"
        # "Update symbols on the listbox"
        n294 = event-data() -> ("PlatMods.Shift"=w490:bool, "Row"=w492:i32)  [unwired: 1 in]
        n295 = case shown="True" w490 {
          tunnel: w492 -> [w496 _]
          tunnel: 1 -> [w495 _]
          frame False {
            n296 = property on="CheckList" class="LstBox (strict)"() -> ("Item Symbols"=w494:i32[])  [unwired: 2 in, 2 out]
            n297 = Replace Array Subset(array=w494, new element=w495, index=w496) -> (w493:i32[])
            n298 = property on="CheckList" class="LstBox (strict)"("Item Symbols"=w493) -> ()  [unwired: 2 in, 2 out]
          }
          frame True {
            w497 = 0 ("Top Row")
            n299 = property on="CheckList" class="LstBox (strict)"() -> ("Number of Rows"=w499:u32)  [unwired: 2 in, 2 out]
            n300 = Initialize Array(0, w499) -> (w498:i32[])
            n301 = property on="CheckList" class="LstBox (strict)"("Top Row"=w497, "Value"=w497, "Item Symbols"=w498) -> ()  [unwired: 2 in, 2 out]
          }
        }
      }
      event "CheckList": Key Down {
        # "Update symbols on the listbox\nLeft and right keys check and uncheck"
        n302 = event-data() -> ("VKey"=w503:T23)  [unwired: 1 in]
        n303 = case shown="\"Left\", \"Right\"" w503 {
          selector: w503 -> [w508 _]
          tunnel: eventvkey."Left" ("VKey") -> [w506 _]
          frame "Left", "Right" {
            n304 = Equal?(x=w506, y=w508) -> (x = y?=w507:bool)
            n305 = Select(t=0, s=w507, f=1) -> (s? t:f=w509:i32)
            n306 = property on="CheckList" class="LstBox (strict)"() -> ("Item Symbols"=w512:i32[])  [unwired: 2 in, 2 out]
            n307 = Replace Array Subset(array=w512, new element=w509, index="CheckList") -> (w511:i32[])
            n308 = property on="CheckList" class="LstBox (strict)"("Item Symbols"=w511) -> ()  [unwired: 2 in, 2 out]
          }
          frame Default {
          }
        }
      }
      event "Motor.Enable": Value Change {
        # "When the test mode otor enable helper is set, update that\ntree row item's value"
        n309 = event-data() -> ("NewVal"=w518:bool)  [unwired: 1 in]
        n310 = Unbundle("Motor") -> ("Value"=w517:dbl)  [unwired: 1 out]
        n311 = Select(t=w517, s=w518, f=0.0) -> (s? t:f=w515:dbl)
        n312 = call <vilib>:"NT Write Number.vi"("Numeric"=w515, "Name"=w514) -> ()  [unwired: 9 in, 1 out]
      }
      event "Test Slider": Value Change {
        # "When the test mode slider helper is set, update that\ntree row item's value"
        n313 = event-data() -> ("NewVal"=w521:dbl)  [unwired: 1 in]
        n314 = call <vilib>:"NT Write Number.vi"("Numeric"=w521, "Name"=w522) -> ()  [unwired: 9 in, 1 out]
      }
      event "On/Off": Value Change {
        # "When the test mode on/off helper value is set, update that\ntree row item's value"
        n315 = event-data() -> ("NewVal"=w526:bool)  [unwired: 1 in]
        n316 = Boolean To (0,1)(Boolean=w526) -> (0, 1=w525:i16)
        n317 = call <vilib>:"NT Write Number.vi"("Numeric"=w525, "Name"=w524) -> ()  [unwired: 9 in, 1 out]
      }
      event "Rev/Fwd": Value Change {
        # "When the test mode helper value for relays is set, update that\ntree row item's value"
        n318 = event-data() -> ("NewVal.Forward"=w534:bool, "NewVal.Reverse"=w533:bool)  [unwired: 1 in]
        n319 = Boolean To (0,1)(Boolean=w534) -> (0, 1=w530:i16)
        n320 = Boolean To (0,1)(Boolean=w533) -> (0, 1=w532:i16)
        n321 = Negate(x=w532) -> (-x=w531:i16)
        n322 = Add(x=w530, y=w531) -> (x+y=w529:i16)
        n323 = call <vilib>:"NT Write Number.vi"("Numeric"=w529, "Name"=w528) -> ()  [unwired: 9 in, 1 out]
      }
      event "Test Ring": Value Change {
        # "When a test mode helper value is selected from the ring,\nset the tree item's variable to the string value"
        n324 = event-data() -> ("NewVal"=w538:u16)  [unwired: 1 in]
        n325 = property on="Test Ring" class="Ring (strict)"() -> ("Strings []"=w539:string[])  [unwired: 2 in, 2 out]
        n326 = Index Array(array=w539, index=w538) -> (element=w537:string)
        n327 = call <vilib>:"NT Write String.vi"("String"=w537, "Name"=w536) -> ()  [unwired: 9 in, 1 out]
      }
      event "Rec Mode": Value Change {
        # "Update globals for recording mode and path to read log from.\nClear when logging and let NetworkTables set path for vision to\nuse."
        n328 = event-data() -> ("NewVal"=w550:enum32{"Stop", "Record", "Playback"})  [unwired: 1 in]
        n329 = global write "WPI_DashboardLogging Global.vi" "Logging Filename"(path "") -> ()
        n330 = global write "WPI_DashboardLogging Global.vi" "Recording"(w550) -> ()
        n331 = case shown="\"Playback\"" w550 {
          tunnel: w549 -> [_ w552 w561]
          tunnel: [_ _ w560] -> w547
          tunnel: [_ _ w559] -> _
          tunnel: w545 -> [_ _ w557]
          tunnel: cluster{i32, i32} {-250, 170} -> [_ _ w556]
          tunnel: [_ _ T24 {"Image Size"=TRUE, "Image Type"=TRUE, "Pixel Value"=TRUE, "ROI Information"=TRUE, "Zoom Factor"=FALSE} ("Image Information Shown:All Elements")] -> w543
          tunnel: [_ _ TRUE ("Zoom Factor")] -> w542
          tunnel: w541 -> [_ _ w553]
          frame Default {
          }
          frame "Stop", "Record" {
            # "Place Window too"
            n332 = invoke class="VI" method="FP.Close"(reference=w552) -> (reference out=w551:refnum<vi>)  [unwired: 2 in, 2 out]
            n333 = invoke class="VI" method="Abort VI"(reference=w551) -> ()  [unwired: 2 in, 3 out]
          }
          frame "Playback" {
            n334 = call "Open Playback Panel.vi"("Offset"=w556, "DB VI Ref"=w557, "Playback in"=w561) -> ("Playback out"=w558:refnum<vi>)  [unwired: 8 in]
            n335 = register-events(w558, w553) -> (reference out=w560:refnum<event-registration>, error out=w559:errorcluster)  [unwired: 2 in]
          }
        }
        n336 = property on="Camera Image" class="ImageControl"("Image Information Shown"=w543, "Image Information Visible"=w542) -> ()  [unwired: 2 in, 2 out]
        n337 = call <vilib>:"WPI_DashboardNT Log FieldName Cache.vi"("Operation"=enum16{"Lookup/Add", "Index", "Clear"}."Clear") -> ()  [unwired: 8 in, 3 out]
      }
      event Panel Close {
        w563 = enum32{"Stop", "Record", "Playback"}."Stop" ("Rec Mode")
        # "Playback window has been closed, abort"
        n338 = event-data() -> ()  [unwired: 1 in, 4 out]
        n339 = local write "Rec Mode"(w563) -> ()
        n340 = global write "WPI_DashboardLogging Global.vi" "Recording"(w563) -> ()
      }
      event Panel Close {
        # "Abort playback window and ourself"
        n341 = event-data() -> ()  [unwired: 1 in, 4 out]
        n342 = invoke class="VI" method="FP.Close"(reference=w567) -> (reference out=w566:refnum<vi>)  [unwired: 2 in, 2 out]
        n343 = invoke class="VI" method="Abort VI"(reference=w566) -> (error out=w565:errorcluster)  [unwired: 2 in, 2 out]
        n344 = invoke class="VI" method="Abort VI"(error in=w565) -> ()  [unwired: 2 in, 3 out]
      }
      event User Event {
        n345 = event-data() -> ("IDs"=w574:cluster{"RPC field ID":u16, "Unique ID":u16}, "String"=w573:string)  [unwired: 1 in]
        n346 = Bundle("IDs"=w574, "String"=w573) -> (w572:T10)  [unwired: 1 in]
        n347 = call <vilib>:"Retrieve RPC Response.vi"("RPC Response"=w572) -> ("Output"=w570:string[][])  [unwired: 10 in]
        n348 = Build Array (concatenate)(w568, w570) -> (w569:string[][])
        n349 = local write "Command Params"(w569) -> ()
        n350 = local write "Cmd Status"("" ("Cmd Status")) -> ()
      }
      event "Tree": Double Click {
        n351 = event-data() -> ("PlatMods"=w578:T27, "Tag"=w577:string)  [unwired: 1 in]
        n352 = Unbundle(w578) -> ("Shift"=w576:bool)  [unwired: 4 out]
        n353 = Not(x=w576) -> (.not. x?=w575:bool)
        n354 = call <vilib>:"NT Update Persistence.vi"("Persistence"=w575, "Name"=w577) -> ()  [unwired: 9 in, 1 out]
      }
    }
  }
  n355 = while {
    tunnel: w64 -> [w581]
    i -> [w584]
    stop <- FALSE stop-if-true
    n356 = Wait (ms)(milliseconds to wait=u32 100) -> ()  [unwired: 1 out]
    n357 = case shown="\"Stop\", Default" "Rec Mode" {
      tunnel: w584 -> [_ _ w599]
      tunnel: [w586 u32 11141120 ("Target Color") w588] -> w580
      frame "Stop", Default {
        # "Reset the color, extra updates don't cost much"
        n358 = call "Alliance Color.vi"() -> ("Alliance Color"=w586:u32)
      }
      frame "Record" {
      }
      frame "Playback" {
        # "Playback"
        n359 = Quotient & Remainder(x=w599, y=u32 50 ("milliseconds to wait")) -> (x-y*floor(x/y)=w595:u32)  [unwired: 1 out]
        n360 = Divide(x=w595, y=u32 50 ("milliseconds to wait")) -> (x/y=w592:dbl)
        n361 = Multiply(x=6.283185307179586, y=w592) -> (x*y=w597:dbl)
        n362 = Sine(x=w597) -> (sin(x)=w596:dbl)
        n363 = Absolute Value(x=w596) -> (abs(x)=w589:dbl)
        n364 = call "Interpolate RGB Color.vi"("Proportion"=w589, "Target Color"=u32 30976, "Base Color"=u32 2829099) -> ("Result Color"=w588:u32)  [unwired: 8 in]
      }
    }
    n365 = property class="Pane"(reference=w581, "PaneColor"=w580) -> ()  [unwired: 1 in, 2 out]
  }
  n366 = local write "Dashboard Tab"(T3."Custom" ("Dashboard Tab")) -> ()
  n367 = property on="On/Off" class="Bool (strict)"("Visible"=w33) -> ()  [unwired: 2 in, 2 out]
  n368 = property on="Motor" class="Clust (strict)"("Visible"=w33) -> ()  [unwired: 2 in, 2 out]
  n369 = property on="Progress" class="Clust (strict)"("Visible"=w33) -> ()  [unwired: 2 in, 2 out]
  n370 = property on="Test Ring" class="Ring (strict)"("Visible"=w33) -> ()  [unwired: 2 in, 2 out]
  n371 = property on="Rev/Fwd" class="Clust (strict)"("Visible"=w33) -> ()  [unwired: 2 in, 2 out]
  n372 = while {
    tunnel: u16 1741 ("timeout ms (25000)") -> [w601]
    stop <- FALSE stop-if-true
    n373 = TCP Create Listener(10:w601) -> (0:w600:errorcluster, 3:w602:refnum<k5>)  [unwired: 4 in, 1 out]
    n374 = case shown="No Error" w600 {
      selector: w600 -> [w604 _]
      tunnel: w602 -> [w605 _]
      frame No Error {
        n375 = while {
          tunnel: w605 -> [w608]
          tunnel: w604 -> [w607]
          stop <- FALSE stop-if-true
          n376 = TCP Wait On Listener(8:w607, 11:w608) -> (0:w609:errorcluster, 4:w610:refnum<k5>)  [unwired: 2 in, 3 out]
          n377 = local write "TCP"(w610) -> ()
          n378 = case shown="No Error" w609 {
            frame No Error {
            }
            frame Error {
              n379 = Wait (ms)(milliseconds to wait=u32 1000) -> ()  [unwired: 1 out]
            }
          }
        }
      }
      frame Error {
        n380 = Wait (ms)(milliseconds to wait=u32 1000) -> ()  [unwired: 1 out]
      }
    }
  }
  n381 = local write "Command Selection"(u16 0 ("milliseconds to wait")) -> ()
  n382 = local write "Command Params"(string[][] [] ("Command Params")) -> ()
  n383 = global write "WPI_DashboardLogging Global.vi" "Recording"(w58) -> ()
  n384 = local write "Rec Mode"(w58) -> ()
  n385 = call <vilib>:"NT Write String.vi"("String"="Select Auto", "Name"="Auto Selector") -> ()  [unwired: 9 in, 1 out]
  n386 = while {
    stop <- FALSE stop-if-true
    n387 = Wait (ms)(milliseconds to wait=500) -> ()  [unwired: 1 out]
    n388 = Random Number (0-1)() -> (number: 0 to 1=w620:dbl)
    n389 = Multiply(x=w620, y=22.0) -> (x*y=w624:dbl)
    n390 = Add(x=w624, y=80.0) -> (x+y=w618:dbl)
    "Steam Power" <- w618
    n391 = Greater Or Equal?(x=w618, y=100.0) -> (x >= y?=w617:bool)
    n392 = property on="String 2" class="Str"("Visible"=w617, "Text.TextColor"=u32 16711680, "Text.FontSize"=40, "Text.FontBold"=TRUE) -> ()  [unwired: 2 in, 2 out]
    "String 2" <- "STEAM OVERLOAD!!!"
  }
